vi "map.to.local.sub.vi"(11 "map in":map{i32, string}(c390)) -> (3 "array out":T1[](array[typedef]))   [LabVIEW 2024, in "manager_daemon.lvclass"]
uses:
  manager_daemon.lvclass
  manager_daemon.lvclass/manager_daemon.ctl
  CV_RESTful_Library/typedefs/cv_issue.generic_credit--cluster.ctl
  CV_RESTful_Library/CV_RESTful_Lib.lvlib
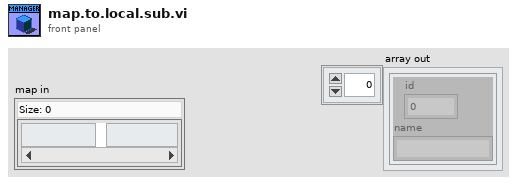
[diagram p1: front panel]
types:
  T1 = typedef "CV_RESTful_Lib.lvlib/cv_issue.generic_credit--cluster.ctl" = cluster{"id":i32, "name":string}
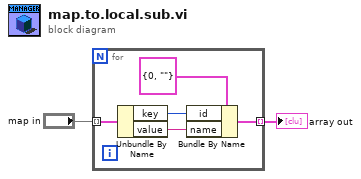
[diagram p0: block diagram]
diagram:
  n1 = for {
    tunnel: "map in" -> [w7] mode=indexing
    tunnel: [w3] -> w1 mode=indexing
    n2 = Unbundle By Name(w7) -> ("key"=w5:i32, "value"=w4:string)
    n3 = Bundle By Name(cluster=T1 {"id"=0, "name"=""} ("character_credit"), "id"=w5, "name"=w4) -> (w3:T1)
  }
  "array out" <- w1
